vi "Reschedule Acquire.vi"(8 "error in (no error)":errorcluster, 10 "Sample Time":i32=1000, 11 "Sensor in":refnum<class "Sensor.lvclass">) -> (0 "error out":errorcluster, 3 "Sensor out":refnum<class "Sensor.lvclass">)   [LabVIEW 2012, in "Sensor Definition.lvlib" / "Sensor.lvclass"]
doc: "Change the update frequency of the sensor.\n\nTime is in ms.\n\nA negative value will stop scheduled updates."
uses:
  Sensor.lvclass
  Sensor.lvclass/Sensor.ctl
  <vilib>/ActorFramework/Time-Delayed Send Message/Time-Delay Override Options.ctl
  Sensor Messages/Acquire Msg/Acquire Msg.lvclass
  <vilib>/ActorFramework/Message Enqueuer/Message Priority.ctl
  <vilib>/ActorFramework/Actor/Actor.lvclass/Actor.ctl
  <vilib>/ActorFramework/Message Enqueuer/Message Enqueuer.lvclass/Message Enqueuer.ctl
  SensorInfo.lvclass/SensorInfo.ctl
  Read Scheduled Delivery Notifier.vi
  Read SensorInfo.vi
  SensorInfo/Write Sample Time.vi
  Write Scheduled Delivery Notifier.vi
  Write SensorInfo.vi
  <vilib>/ActorFramework/Message Enqueuer/Init from Existing Queue.vi
  SensorInfo.lvclass
  <vilib>/ActorFramework/Message Enqueuer/Message Enqueuer.lvclass
  Win8uiFramework/Win8uiFramework.lvlib
  <vilib>/ActorFramework/Actor/Actor.lvclass
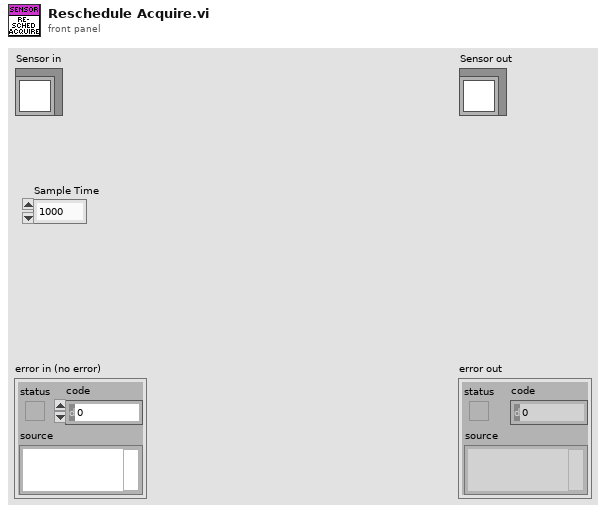
[diagram p1: front panel]
types:
  T1 = typedef "Actor Framework.lvlib/Message Enqueuer.lvclass/Message Priority.ctl" = enum16{"Low", "Normal", "High"}
  T2 = typedef "Time-Delay Override Options.ctl" = enum16{"Send next copy now", "Skip next scheduled copy", "Send next copy now and stop all further copies", "Stop all further copies"}
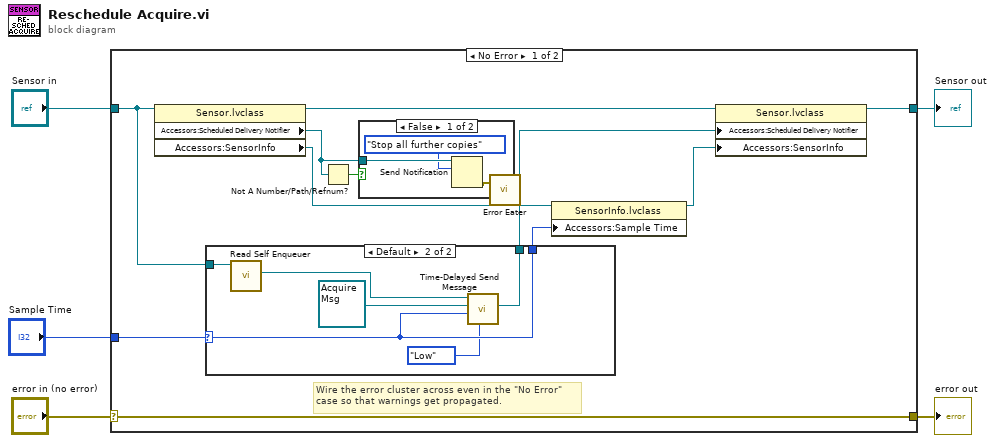
[diagram p0: block diagram]
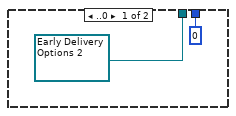
[diagram p2: hidden frame]
diagram:
  n1 = case shown="No Error" "error in (no error)" {
    selector: "error in (no error)" -> [w16 w29]
    tunnel: [w16 w29] -> w4
    tunnel: [w15 w28] -> w2
    tunnel: "Sensor in" -> [w14 w28]
    tunnel: "Sample Time" -> [w9 _]
    frame No Error {
      # "Wire the error cluster across even in the \"No Error\"\ncase so that warnings get propagated."
      n2 = property class="Sensor.lvclass"(reference=w14) -> (reference out=w13:refnum<class "Sensor.lvclass">, "Accessors:Scheduled Delivery Notifier"=w11:refnum<notifier>, "Accessors:SensorInfo"=w8:refnum<class "SensorInfo.lvclass">)  [unwired: 1 in, 1 out]
      n3 = case shown="Default" w9 {
        selector: w9 -> [_ w20]
        tunnel: w14 -> [_ w24]
        tunnel: [w18 w23] -> w10
        tunnel: [0 ("Sample Time") w20] -> w7
        frame ..0 {
          w18 = refnum<notifier> refnum items=["Send next copy now", "Skip next scheduled copy", "Send next copy now and stop all further copies", "Stop all further copies"] ("Delivery Notifier")
        }
        frame Default {
          n4 = call <vilib>:"Read Self Enqueuer.vi"("Actor"=w24) -> ("Self Enqueuer"=w21:refnum<class "Message Enqueuer.lvclass">)  [unwired: 10 in]
          n5 = call <vilib>:"Time-Delayed Send Message.vi"("Message Priority (Normal)"=Message_Priority."Low", "Milliseconds To Wait"=w20, "Message"=refnum<class "Acquire Msg.lvclass"> refnum ("Sensor Definition.lvlib:Acquire Msg.lvclass"), "Message Enqueuer"=w21) -> ("Delivery Notifier"=w23:refnum<notifier>)  [unwired: 6 in, 1 out]
        }
      }
      n6 = Not A Number/Path/Refnum?(number/path/refnum=w11) -> (NaN/Path/Refnum?=w12:bool)
      n7 = case shown="False" w12 {
        tunnel: w11 -> [w27 _]
        frame False {
          n8 = Send Notification(notification=Time-Delay_Override_Options."Stop all further copies", notifier=w27) -> (error out=w25:errorcluster)  [unwired: 1 in, 1 out]
          n9 = call "Error Eater.vi"("error in (no error)"=w25) -> ()  [unwired: 2 in]
        }
        frame True {
        }
      }
      n10 = property class="SensorInfo.lvclass"(reference=w8, "Accessors:Sample Time"=w7) -> (reference out=w6:refnum<class "SensorInfo.lvclass">)  [unwired: 1 in, 1 out]
      n11 = property class="Sensor.lvclass"(reference=w13, "Accessors:Scheduled Delivery Notifier"=w10, "Accessors:SensorInfo"=w6) -> (reference out=w15:refnum<class "Sensor.lvclass">)  [unwired: 1 in, 1 out]
    }
    frame Error {
    }
  }
  "error out" <- w4
  "Sensor out" <- w2
